vi "DB- User Management.vi"(6 "Enum":T1(ring), 8 "error in (no error)":errorcluster, 10 "Input data":T2, 11 "DB Path":path) -> (0 "error out":errorcluster, 3 "Data Read":variant[][](array[variant]))   [LabVIEW 2014]
uses:
  <vilib>/addons/database/Connection.llb/DB Tools Open Connec (Path).vi
  <vilib>/addons/database/NI_Database_API.lvlib
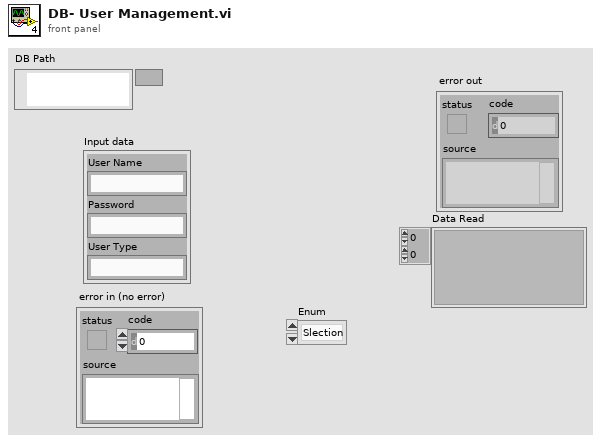
[diagram p1: front panel]
types:
  T1 = enum16{"Slection", "Insertdata", "Edit/Upload", "DB-Read", "Delete"}
  T2 = cluster{"User Name":string, "Password":string, "User Type":string}
  T3 = typedef "NI_Database_API.lvlib/Conn ObjectReference.ctl" = refnum<k1>
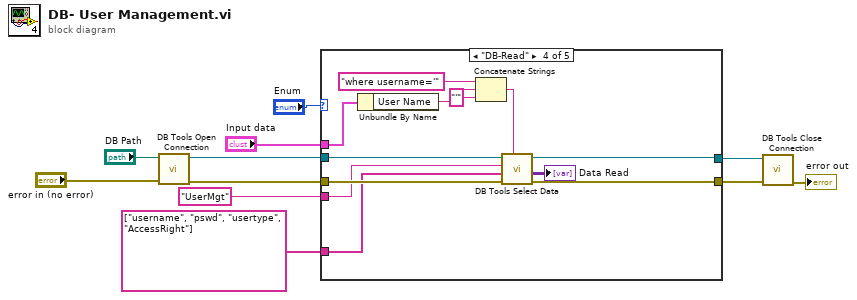
[diagram p0: block diagram]
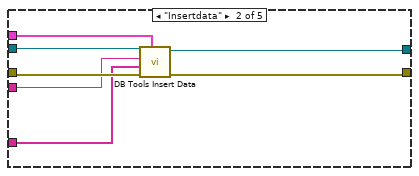
[diagram p3: hidden frame]
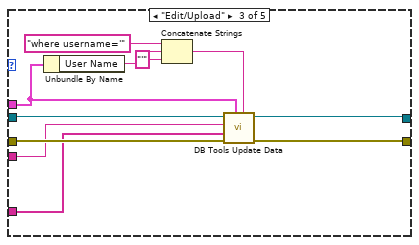
[diagram p4: hidden frame]
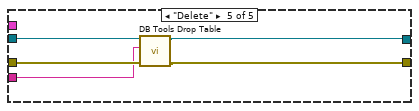
[diagram p5: hidden frame]
diagram:
  n1 = call-poly <vilib>:"DB Tools Open Connection.vi"("error in (no error)"="error in (no error)", "connection information"="DB Path") -> ("error out"=w3:errorcluster, "connection reference"=w2:T3)  [unwired: 6 in]
  n2 = case shown="\"DB-Read\"" "Enum" {
    tunnel: w2 -> [w13 w20 w31 w43 w48]
    tunnel: w3 -> [w12 w19 w30 w42 w47]
    tunnel: [w13 w18 w24 w34 w45] -> w6
    tunnel: [w12 w17 w23 w33 w44] -> w5
    tunnel: "Input data" -> [_ w14 w25 w36 _]
    tunnel: string[] ["username", "pswd", "usertype", "AccessRight"] ("columns") -> [_ w15 w22 w40 _]
    tunnel: "UserMgt" ("table") -> [_ w16 w21 w41 w46]
    frame "Slection", Default {
    }
    frame "Insertdata" {
      n3 = call <vilib>:"DB Tools Insert Data.vi"("data"=w14, "error in (no error)"=w19, "columns"=w15, "table"=w16, "connection reference"=w20) -> ("error out"=w17:errorcluster, "connection reference out"=w18:T3)  [unwired: 5 in]
    }
    frame "Edit/Upload" {
      n4 = Unbundle By Name(w25) -> ("User Name"=w28:string)
      n5 = Concatenate Strings("where username='" ("condition"), w28, "'" ("User Name")) -> (w26:string)
      n6 = call <vilib>:"DB Tools Update Data.vi"("condition"=w26, "data"=w25, "error in (no error)"=w30, "columns"=w22, "table"=w21, "connection reference"=w31) -> ("error out"=w23:errorcluster, "connection reference out"=w24:T3)  [unwired: 4 in]
    }
    frame "DB-Read" {
      n7 = Unbundle By Name(w36) -> ("User Name"=w38:string)
      n8 = Concatenate Strings("where username='" ("condition"), w38, "'" ("User Name")) -> (w35:string)
      n9 = call <vilib>:"DB Tools Select Data.vi"("condition"=w35, "error in (no error)"=w42, "columns"=w40, "table"=w41, "connection reference"=w43) -> ("error out"=w33:errorcluster, "data"=→"Data Read":variant[][], "connection reference out"=w34:T3)  [unwired: 1 in]
    }
    frame "Delete" {
      n10 = call <vilib>:"DB Tools Drop Table.vi"("error in (no error)"=w47, "table"=w46, "connection reference"=w48) -> ("error out"=w44:errorcluster, "connection reference out"=w45:T3)  [unwired: 5 in]
    }
  }
  n11 = call <vilib>:"DB Tools Close Connection.vi"("error in (no error)"=w5, "connection reference"=w6) -> ("error out"=→"error out":errorcluster)  [unwired: 5 in]
